vi "Load Help File.vi"(8 "error in (no error)":errorcluster, 9 "HTML File to Load":string="MainPage_J1939.html", 11 "Browser":refnum<k7>(container)) -> (0 "error out":errorcluster)   [LabVIEW 2021, in "Software Multi-Plex System Explorer.lvlib"]
doc: "Loads the specified HTML page from the CHM into the browser"
uses:
  Software Multi-Plex System Explorer.lvlib
  <vilib>/Utility/LVLibp/NI_PackedLibraryUtility.lvlib
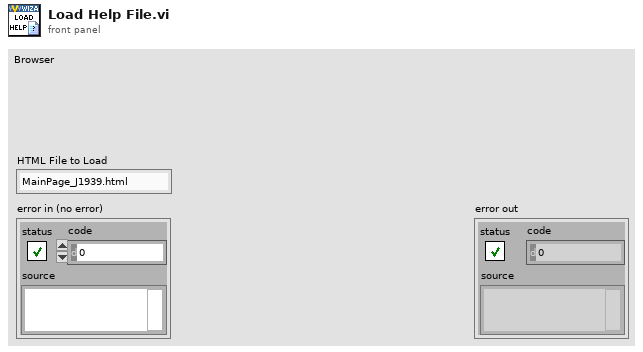
[diagram p1: front panel]
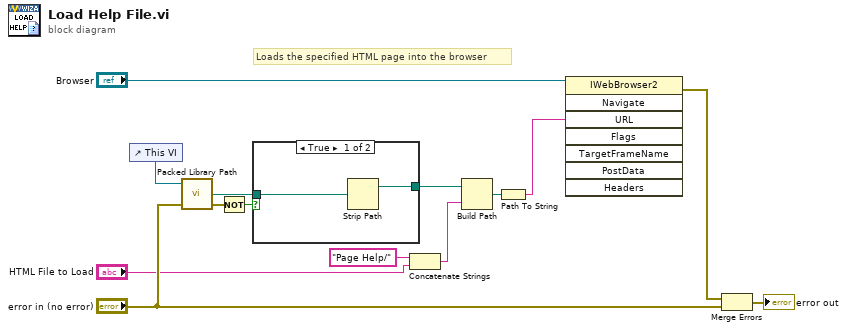
[diagram p0: block diagram]
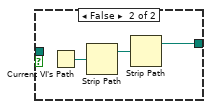
[diagram p2: hidden frame]
diagram:
  # "Loads the specified HTML page into the browser"
  n1 = control-ref of="This VI"() -> (w12:refnum<vi>)
  n2 = call <vilib>:"Packed Library Path.vi"("error in (no error)"="error in (no error)", "vi reference"=w12) -> ("error out"=w9:errorcluster, "packed library path"=w11:path)  [unwired: 1 in, 1 out]
  n3 = Not(x=w9) -> (.not. x?=w10:bool)
  n4 = case shown="True" w10 {
    tunnel: w11 -> [w16 _]
    tunnel: [w15 w17] -> w2
    frame True {
      n5 = Strip Path(path=w16) -> (stripped path=w15:path)  [unwired: 1 out]
    }
    frame False {
      n6 = Current VI's Path() -> (path=w19:path)
      n7 = Strip Path(path=w19) -> (stripped path=w18:path)  [unwired: 1 out]
      n8 = Strip Path(path=w18) -> (stripped path=w17:path)  [unwired: 1 out]
    }
  }
  n9 = Concatenate Strings("Page Help/" ("string"), "HTML File to Load") -> (w4:string)
  n10 = Build Path(base path=w2, name or relative path=w4) -> (appended path=w5:path)
  n11 = Path To String(path=w5) -> (string=w1:string)
  n12 = invoke class="IWebBrowser2" method="Navigate"(reference="Browser", "URL"=w1) -> (error out=w8:errorcluster)  [unwired: 6 in, 7 out]
  n13 = Merge Errors(w8, "error in (no error)") -> (→"error out":errorcluster)
